vi "Read Decimation Channel.vi"(8 "error in":errorcluster, 10 "default decimation":i32=1, 11 "decimation reference in":T1 format="%.0x") -> (0 "error out":errorcluster, 3 "decimation":i32)   [LabVIEW 2027, in "Embedded Data Logger Engine.lvlib"]
uses:
  Embedded Data Logger Engine.lvlib
  <vilib>/NI VeriStand/Custom Device API/Data Reference.ctl
  <vilib>/NI VeriStand/Custom Device API/Global Data Refs.vi
  <vilib>/NI VeriStand/Custom Device API/Custom Device API.lvlib
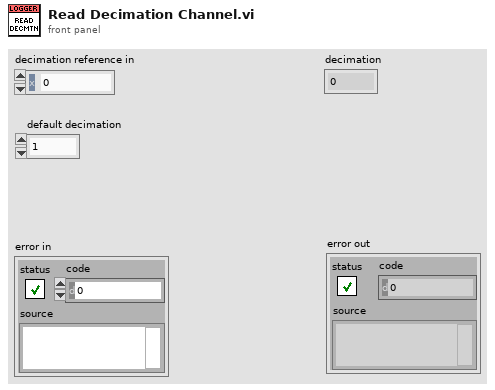
[diagram p1: front panel]
types:
  T1 = typedef "Custom Device API.lvlib/Data Reference.ctl" = i32
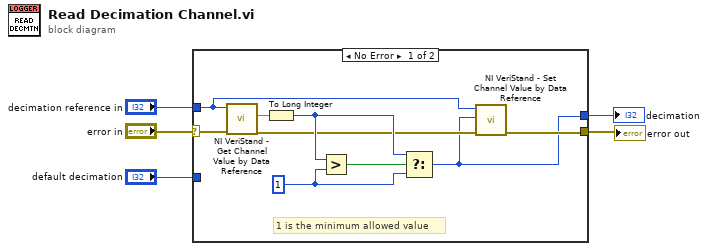
[diagram p0: block diagram]
diagram:
  n1 = case shown="No Error" "error in" {
    selector: "error in" -> [w14 w16]
    tunnel: "decimation reference in" -> [w9 _]
    tunnel: "default decimation" -> [_ w15]
    tunnel: [w6 w15] -> w3
    tunnel: [w7 w16] -> w2
    frame No Error {
      w12 = 1 ("y")
      # "1 is the minimum allowed value"
      n2 = call <vilib>:"NI VeriStand - Get Channel Value by Data Reference.vi"("error in (no error)"=w14, "Data Reference in"=w9) -> ("error out"=w8:errorcluster, "Value"=w11:dbl)  [unwired: 8 in]
      n3 = To Long Integer(number=w11) -> (32bit integer=w10:i32)
      n4 = Greater?(x=w10, y=w12) -> (0:w13:bool)
      n5 = Select(t=w10, s=w13, f=w12) -> (s? t:f=w6:i32)
      n6 = call <vilib>:"NI VeriStand - Set Channel Value by Data Reference.vi"("error in (no error)"=w8, "Value"=w6, "Data Reference in"=w9) -> ("error out"=w7:errorcluster)  [unwired: 8 in]
    }
    frame Error {
    }
  }
  "decimation" <- w3
  "error out" <- w2
